vi "Make Request.vi"(8 "error in (no error)":errorcluster, 9 "Parameters":T2[](array[typedef]), 10 "url":string, 11 "Refnum in":T1) -> (0 "error out":errorcluster, 1 "body":string, 2 "headers":string, 3 "client handle out":T1)   [LabVIEW 2015]
uses:
  <vilib>/httpClient/ClientHandle.ctl
  GET Parameter.ctl
  <vilib>/httpClient/LabVIEWHTTPClient.lvlib
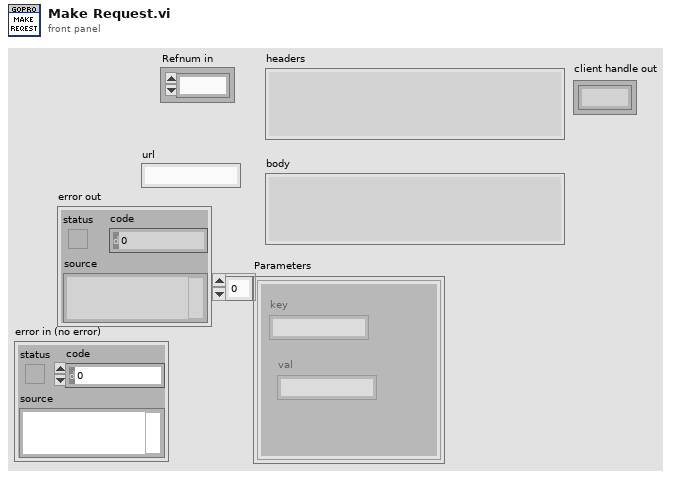
[diagram p1: front panel]
types:
  T1 = typedef "LabVIEWHTTPClient.lvlib/ClientHandle.ctl" = refnum<k1>
  T2 = typedef "GET Parameter.ctl" = cluster{"key":string, "val":string}
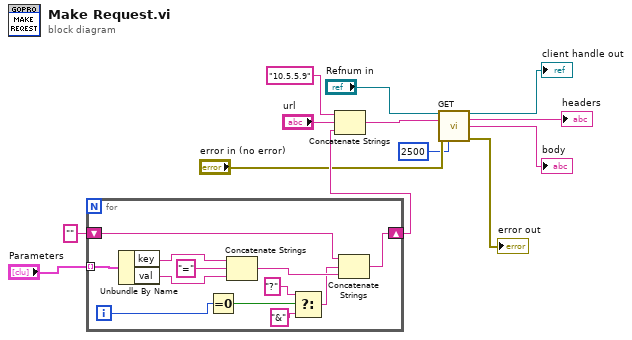
[diagram p0: block diagram]
diagram:
  n1 = for {
    tunnel: "Parameters" -> [w25] mode=indexing
    shift-right: [w14] -> w6
    shift-left: "" -> [w17]
    i -> [w21]
    n2 = Unbundle By Name(w25) -> ("key"=w24:string, "val"=w22:string)
    n3 = Equal To 0?(x=w21) -> (x = 0?=w20:bool)
    n4 = Concatenate Strings(w24, "=", w22) -> (w16:string)
    n5 = Select(t="?", s=w20, f="&") -> (s? t:f=w15:string)
    n6 = Concatenate Strings(w17, w15, w16) -> (w14:string)
  }
  n7 = Concatenate Strings("10.5.5.9", "url", w6) -> (w11:string)
  n8 = call <vilib>:"GET.vi"("client handle"="Refnum in", "url"=w11, "error in (no error)"="error in (no error)", "timeout (10000)"=2500) -> ("client handle out"=→"client handle out":T1, "headers"=→"headers":string, "body"=→"body":string, "error out"=→"error out":errorcluster)  [unwired: 8 in]
